vi "_multiply value.vi"(6 "label":T1, 8 "error in (no error)":errorcluster, 10 "B":refnum<class "Value.lvclass">, 11 "A":refnum<class "Value.lvclass">) -> (0 "error out":errorcluster, 2 "C":refnum<class "Value.lvclass">, 3 "A out":refnum<class "Value.lvclass">)   [LabVIEW 2023, in "LabGRAD.lvlib" / "Value.lvclass"]
uses:
  Value.lvclass
  UiObjects/string control.ctl
  operation.ctl
  Value.lvclass/Value.ctl
  UiObjects/UiObjects.lvclass
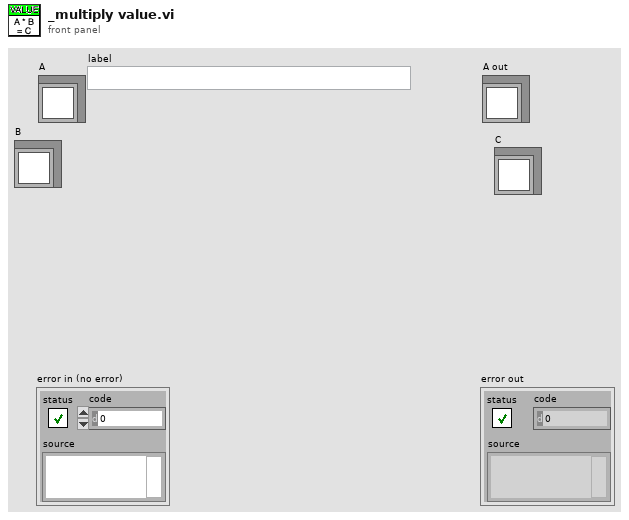
[diagram p1: front panel]
types:
  T1 = typedef "UiObjects.lvlib/UiObjects.lvclass/string control.ctl" = string
  T2 = typedef "LabGRAD.lvlib/Value.lvclass/operation.ctl" = enum16{"nop", "add", "subtract", "power", "multiply", "divide", "tanh"}
  T3 = typedef "UiObjects.lvlib/UiObjects.lvclass/numeric value control.ctl" = dbl
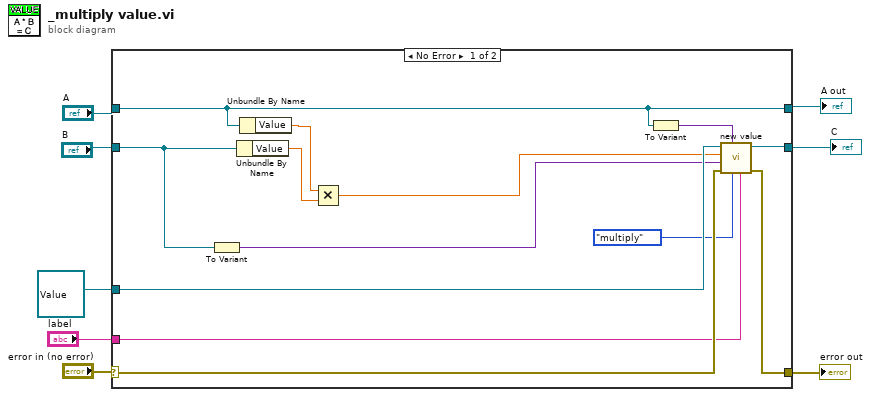
[diagram p0: block diagram]
diagram:
  n1 = case shown="No Error" "error in (no error)" {
    selector: "error in (no error)" -> [w13 w24]
    tunnel: [w12 w24] -> w5
    tunnel: [w19 w23] -> w6
    tunnel: "A" -> [w19 w23]
    tunnel: "B" -> [w18 _]
    tunnel: [w17 w22] -> w2
    tunnel: refnum<class "Value.lvclass"> refnum ("B") -> [w16 w22]
    tunnel: "label" -> [w10 _]
    frame No Error {
      n2 = To Variant(anything=w18) -> (Variant=w15:variant)
      n3 = Unbundle By Name(w18) -> ("Value"=w20:T3)
      n4 = Unbundle By Name(w19) -> ("Value"=w21:T3)
      n5 = Multiply(x=w21, y=w20) -> (x*y=w14:T3)
      n6 = To Variant(anything=w19) -> (Variant=w9:variant)
      n7 = call "new value.vi"("Label"=w10, "operation"=operation."multiply", "Previous"=w9, "error in (no error)"=w13, "Other"=w15, "data"=w14, "Value in"=w16) -> ("error out"=w12:errorcluster, "Value out"=w17:refnum<class "Value.lvclass">)  [unwired: 3 in]
    }
    frame Error {
    }
  }
  "error out" <- w5
  "A out" <- w6
  "C" <- w2
